vi "Send Update DT Event.vi"(7 "Message Priority (Normal)":T3=enum."Normal", 8 "error in (no error)":errorcluster, 10 "event data":T1, 11 "Message Enqueuer":refnum<class "Message Enqueuer.lvclass">) -> (0 "error out":errorcluster, 3 "Message Enqueuer out":refnum<class "Message Enqueuer.lvclass">)   [LabVIEW 2016, in "Controller UI.lvlib" / "Update DT Event Msg.lvclass"]
doc: "This VI sends the message to an actor."
uses:
  <userlib>/Common Components/Controller UI Messages/Update DT Event Msg/Update DT Event Msg.lvclass
  <vilib>/ActorFramework/Message Enqueuer/Message Enqueuer.lvclass
  <vilib>/ActorFramework/Message Enqueuer/Message Priority.ctl
  <userlib>/Common Components/Controller UI/Update DT event data.ctl
  <userlib>/Common Components/Controller UI/Update DT Cmd.ctl
  C:/Program Files (x86)/National Instruments/LabVIEW 2016/vi.lib/ActorFramework/Message/Message.lvclass
  <userlib>/Common Components/Controller UI Messages/Update DT Event Msg/Update DT Event Msg.lvclass/Update DT Event Msg.ctl
  <vilib>/ActorFramework/Message Enqueuer/Message Enqueuer.lvclass/Message Enqueuer.ctl
  <vilib>/ActorFramework/Message Priority Queue/Priority Enqueue.vi
  <userlib>/Common Components/Controller UI/Controller UI.lvclass
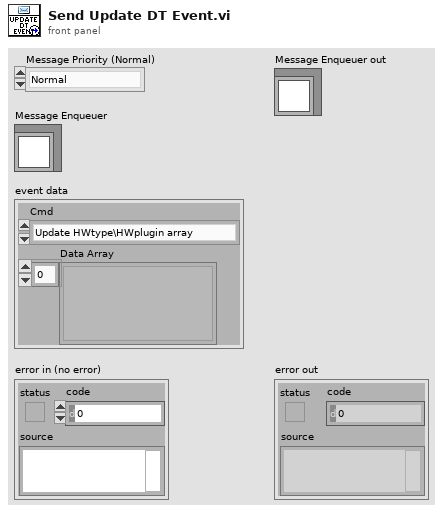
[diagram p1: front panel]
types:
  T1 = typedef "Controller UI.lvlib/Controller UI.lvclass/Update DT event data.ctl" = cluster{"Cmd":T2, "Data Array":variant[]}
  T2 = typedef "Controller UI.lvlib/Controller UI.lvclass/Update DT Cmd.ctl" = enum16{"Update HWtype\\HWplugin array", "Update Checked-out", "Update COMM Status", "Load DevInfo from File", "Save DevInfo to File", "Update COMM Address List"}
  T3 = typedef "Actor Framework.lvlib/Message Enqueuer.lvclass/Message Priority.ctl" = enum16{"Low", "Normal", "High"}
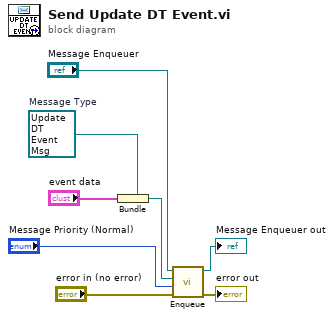
[diagram p0: block diagram]
diagram:
  w5 = refnum<class "Update DT Event Msg.lvclass"> refnum  # Message Type
  n1 = Bundle(cluster=w5, "event data") -> (w4:refnum<class "Update DT Event Msg.lvclass">)
  n2 = call <vilib>:"Enqueue.vi"("error in (no error)"="error in (no error)", "Message Priority (Normal)"="Message Priority (Normal)", "Message"=w4, "Message Enqueuer in"="Message Enqueuer") -> ("error out"=→"error out":errorcluster, "Message Enqueuer out"=→"Message Enqueuer out":refnum<class "Message Enqueuer.lvclass">)  [unwired: 6 in]
